vi "NGDUTCheck.vi"(11 "YTESTER测试数据":T1 caption="不要修改！") -> (3 "YTESTER结论":T2)   [LabVIEW 2017]
doc: "VIDescription=不合格金机点检，此Step一定要放最后，会根据前面的测试结果判断点检品点检是否正确！"
uses:
  YtCommon.lvlibp/yt`Step StepBaseInput.ctl
  YtCommon.lvlibp/yt`Step StepResult.ctl
  YtCommon.lvlibp/yt`Step TestData.ctl
  YtCommon.lvlibp/yt`Step System Queue.ctl
  Step`s VIs/YYLLGeneric/variable_W.ctl
  YtCommon.lvlibp/yt`Data-Ytester Type Data.ctl
  9b849966-5727-4c2c-94ee-55c4a0c550b3.vi
  573427c3-80ef-4845-b534-6c56ed2aebbb.vi
  <vilib>/Utility/error.llb/Clear Errors.vi
  YtCommon.lvlibp/yt`varSystemlib IO Read Variable.vi
  YtCommon.lvlibp
panel:
  in  "YTESTER开放参数":T4={"YTESTER_BaseInput"={"isTest"=TRUE, "isSkip"=FALSE, "StepName"="NG不合格金机点检", "OnPass"=enum."Next", "OnFail"=enum."Terminate", "ReTestNumber"=0.0}, "不合格点检品SN"=[], "点检有效时间（小时）"=24.0}
  # "NG不合格品点检检查"
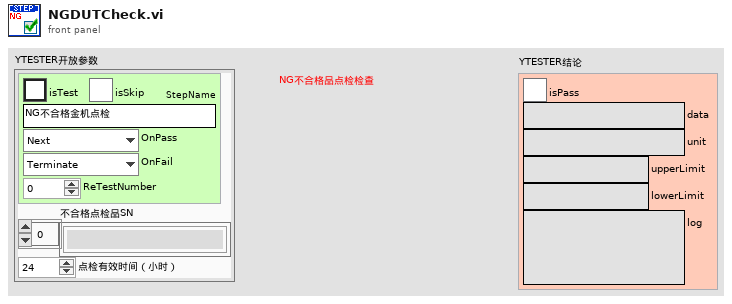
[diagram p1: front panel]
types:
  T1 = typedef "YtCommon.lvlibp/yt`Step TestData.ctl" = cluster{"Socket(From1)":i32, "SN":refnum<notifier>, "StopFlagRef":refnum<notifier>, "YT System Queue":refnum<queue>}
  T2 = typedef "YtCommon.lvlibp/yt`Step StepResult.ctl" = cluster{"isPass":bool, "data":string, "unit":string, "upperLimit":string, "lowerLimit":string, "log":string}
  T3 = typedef "YtCommon.lvlibp/yt`Step StepBaseInput.ctl" = cluster{"isTest":bool, "isSkip":bool, "StepName":string, "OnPass":enum16{"Next", "ToOVER", "Terminate"}, "OnFail":enum16{"Next", "ToOVER", "Terminate"}, "ReTestNumber":dbl}
  T4 = cluster{"YTESTER_BaseInput":T3, "不合格点检品SN":string[], "点检有效时间（小时）":dbl}
  T5 = typedef "variable_W.ctl" = cluster{"YT_TYPE":T6, "TypeData":string[], "Tips":string}
  T6 = typedef "YtCommon.lvlibp/yt`Data-Ytester Type Data.ctl" = enum16{"NULL", "NUM", "BOOL", "TXT", "ENUM", "TIME", "PATH", "VISA", "COMBO", "ColorBox", "RadioBtn", "Array_NUM", "Array_BOOL", "Array_TXT", "Array_ENUM", "Array_PATH", "Array_COMBO"}
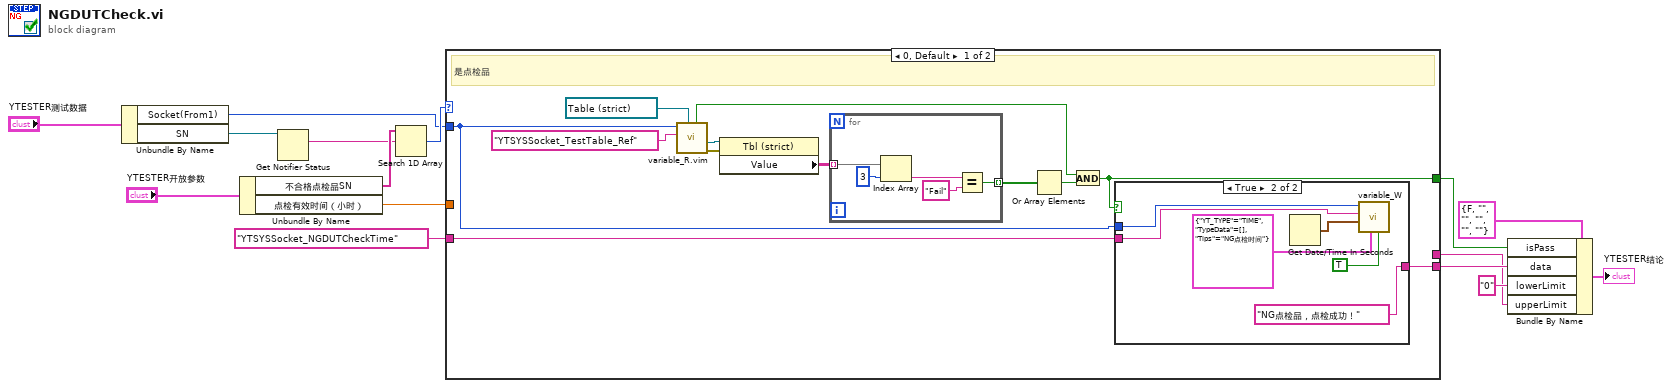
[diagram p0: block diagram]
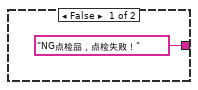
[diagram p2: hidden frame]
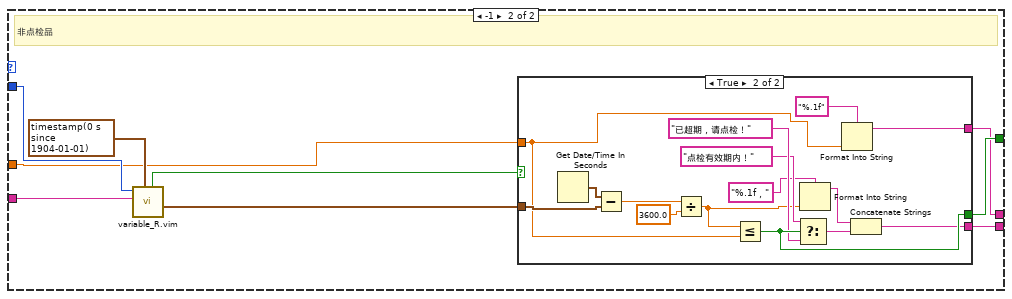
[diagram p3: hidden frame]
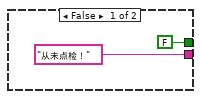
[diagram p4: hidden frame]
diagram:
  n1 = Unbundle By Name("YTESTER测试数据") -> ("Socket(From1)"=w7:i32, "SN"=w11:refnum<notifier>)
  n2 = Unbundle By Name("YTESTER开放参数") -> ("不合格点检品SN"=w10:string[], "点检有效时间（小时）"=w3:dbl)
  n3 = Get Notifier Status(notifier=w11) -> (current notification=w9:string)  [unwired: 1 in, 4 out]
  n4 = Search 1D Array(1D array=w10, element=w9) -> (index of element=w8:i32)  [unwired: 1 in]
  n5 = case shown="0, Default" w8 {
    tunnel: w7 -> [w21 w48]
    tunnel: [w27 w44] -> w6
    tunnel: [w18 w43] -> w5
    tunnel: "YTSYSSocket_NGDUTCheckTime" ("format string") -> [w26 w47]
    tunnel: w3 -> [_ w41]
    tunnel: [_ w40] -> w1
    frame 0, Default {
      # "是点检品"
      n6 = call "variable_R.vim"("type"=refnum<vi> refnum ("TestTable"), "待获取变量名称"="YTSYSSocket_TestTable_Ref", "函数池名称"=w21) -> ("error out"=w22:errorcluster, "value"=w23:refnum<vi>, "found?"=w20:bool)  [unwired: 4 in, 2 out]
      n7 = property class="Tbl (strict)"(reference=w23, error in=w22) -> ("Value"=w17:string[][])  [unwired: 2 out]
      n8 = for {
        tunnel: w17 -> [w31] mode=indexing
        tunnel: [w28] -> w16 mode=indexing
        n9 = Index Array(array=w31, index=3) -> (element=w29:string)
        n10 = Equal?(x=w29, y="Fail") -> (x = y?=w28:bool)
      }
      n11 = Or Array Elements(Boolean array=w16) -> (logical OR=w19:bool)
      n12 = And(x=w20, y=w19) -> (x .and. y?=w18:bool)
      n13 = case shown="True" w18 {
        tunnel: w21 -> [_ w39]
        tunnel: ["NG点检品，点检失败！" "NG点检品，点检成功！"] -> w27
        tunnel: w26 -> [_ w35]
        frame False {
        }
        frame True {
          n14 = Get Date/Time In Seconds() -> (seconds since 1Jan1904=w37:timestamp)
          n15 = call "variable_W.vi"("永久生成在本地（F）"=TRUE, "附加的Information"=T5 {"YT_TYPE"=enum."TIME", "TypeData"=[], "Tips"="NG点检时间"}, "待写入池的输入控件"=w37, "待写入池变量名称"=w35, "函数池名称 in"=w39) -> ()  [unwired: 4 in, 3 out]
        }
      }
    }
    frame -1 {
      # "非点检品"
      n16 = call "variable_R.vim"("type"=timestamp(0 s since 1904-01-01), "待获取变量名称"=w47, "函数池名称"=w48) -> ("value"=w42:timestamp, "found?"=w45:bool)  [unwired: 4 in, 3 out]
      n17 = case shown="True" w45 {
        tunnel: ["从未点检！" w52] -> w44
        tunnel: [FALSE w58] -> w43
        tunnel: w42 -> [_ w64]
        tunnel: w41 -> [_ w60]
        tunnel: [_ w59] -> w40
        frame False {
        }
        frame True {
          n18 = Get Date/Time In Seconds() -> (seconds since 1Jan1904=w65:timestamp)
          n19 = Subtract(x=w65, y=w64) -> (x-y=w63:dbl)
          n20 = Divide(x=w63, y=3600.0 ("x")) -> (x/y=w53:dbl)
          n21 = Less Or Equal?(x=w53, y=w60) -> (x <= y?=w58:bool)
          n22 = Select(t="点检有效期内！", s=w58, f="已超期，请点检！") -> (s? t:f=w56:string)
          n23 = Format Into String(format string="%.1f，", w53) -> (resulting string=w51:string)  [unwired: 2 in, 1 out]
          n24 = Format Into String(format string="%.1f", w60) -> (resulting string=w59:string)  [unwired: 2 in, 1 out]
          n25 = Concatenate Strings(w51, w56) -> (w52:string)
        }
      }
    }
  }
  n26 = Bundle By Name(cluster=T2 {"isPass"=FALSE, "data"="", "unit"="", "upperLimit"="", "lowerLimit"="", "log"=""} ("Result"), "isPass"=w5, "data"=w6, "lowerLimit"="0", "upperLimit"=w1) -> (→"YTESTER结论":T2)
